vi "Header Names Single.vi"(11 "Dynamic Data":dynamicdata(waveform)) -> (3 "Signals Out":dynamicdata(waveform))   [LabVIEW 2017]
uses:
  <vilib>/express/express shared/transition.llb/Dynamic To Waveform Array.vi
  <vilib>/express/express signal manip/GetorSetDDTAttributes/Set DDT Attributes/SetT0.vi
  <vilib>/express/express shared/transition.llb/Waveform Array To Dynamic.vi
  <vilib>/express/express signal manip/GetorSetDDTAttributes/Set DDT Attributes/Set DDT Properties.xnode
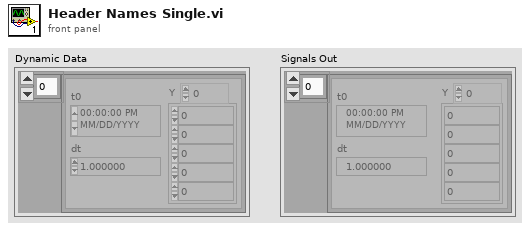
[diagram p1: front panel]
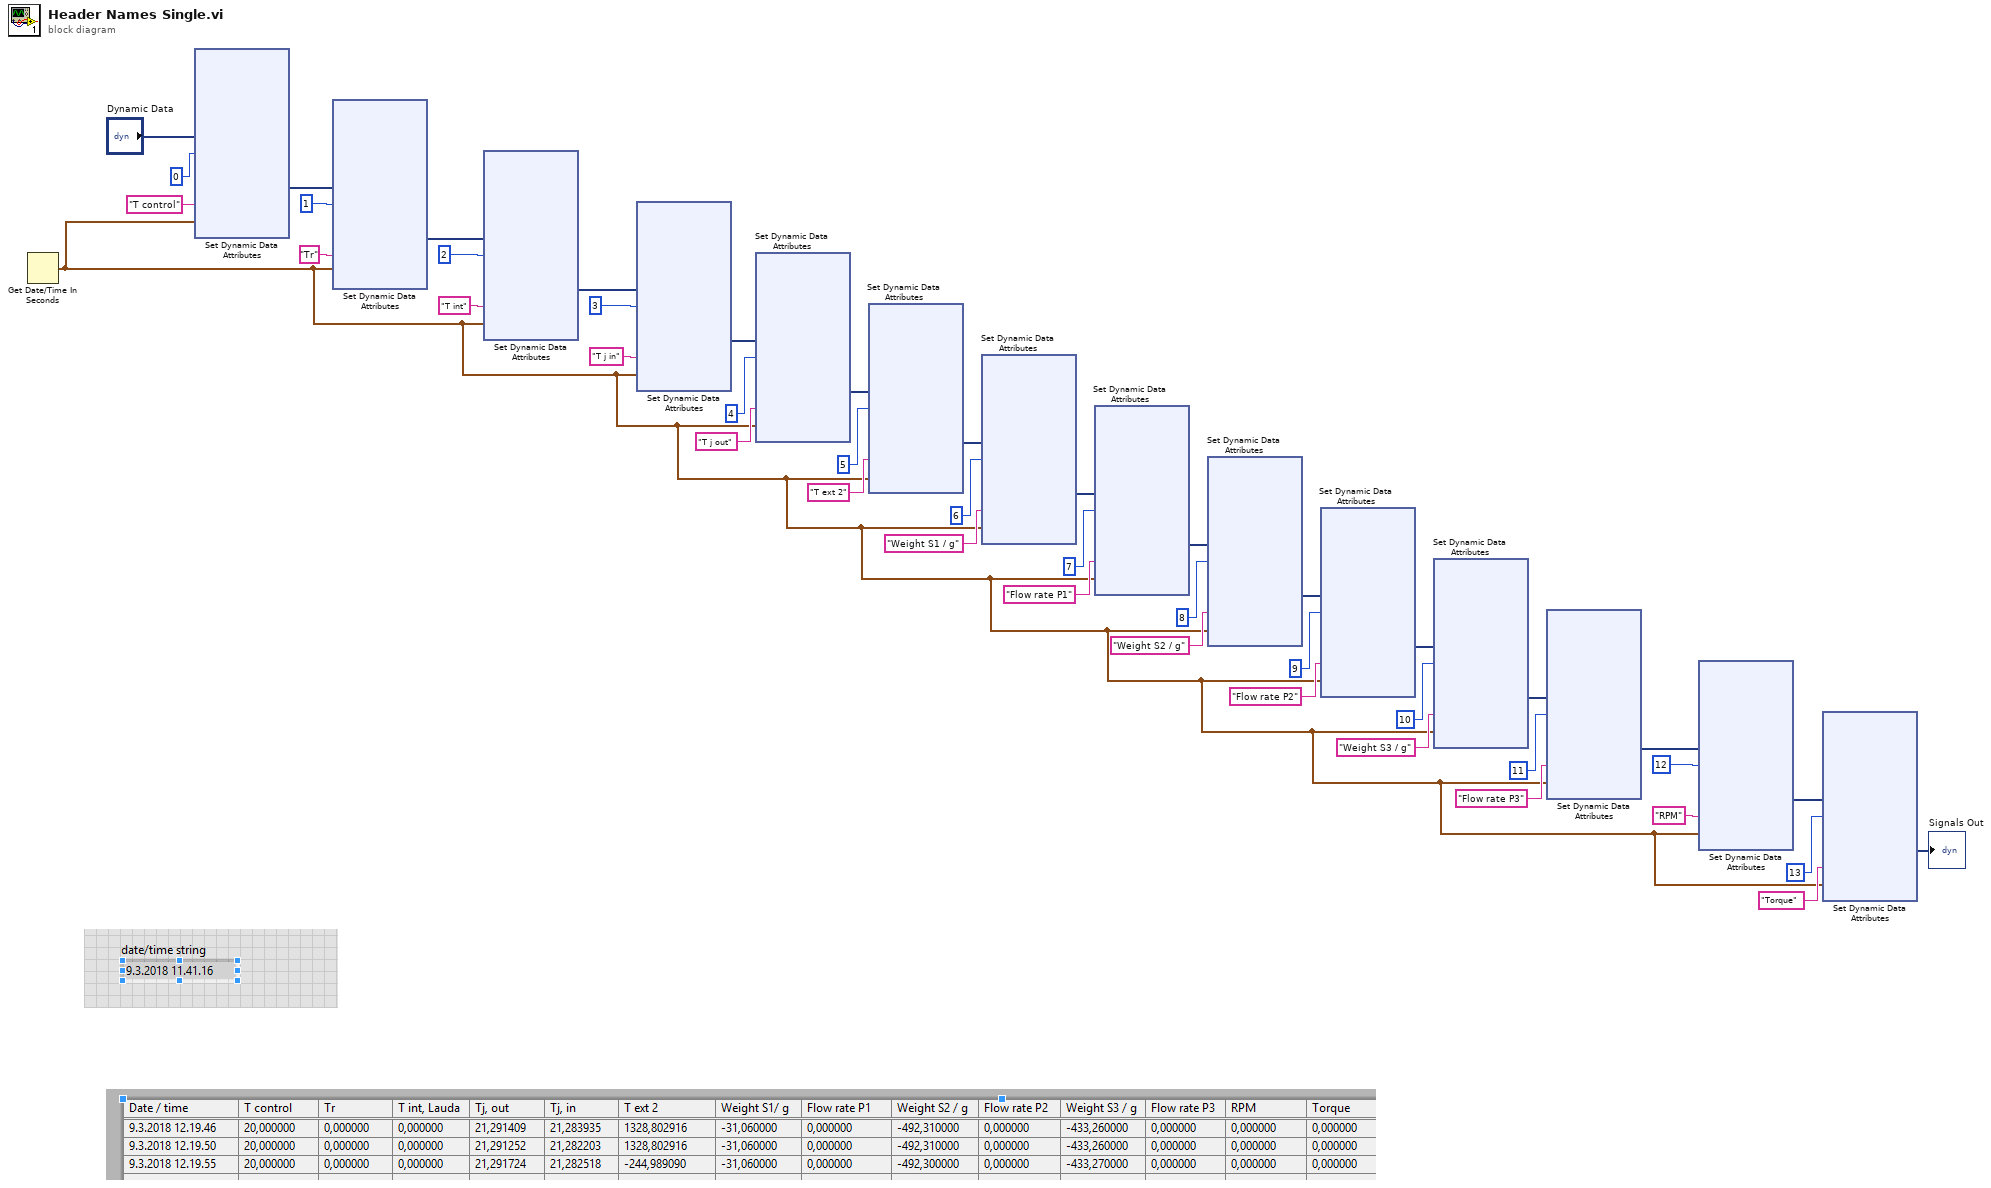
[diagram p0: block diagram]
diagram:
  n1 = Get Date/Time In Seconds() -> (seconds since 1Jan1904=w1:timestamp)
  n2 = xnode "Set Dynamic Data Attributes"("Signals In"="Dynamic Data", "Signal Index"=0, "Signal Name"="T control", "Timestamp"=w1) -> ("Signals Out"=w10:dynamicdata)  [unwired: 1 in, 1 out]
  n3 = xnode "Set Dynamic Data Attributes"("Signals In"=w10, "Signal Index"=1, "Signal Name"="Tr", "Timestamp"=w1) -> ("Signals Out"=w11:dynamicdata)  [unwired: 1 in, 1 out]
  n4 = xnode "Set Dynamic Data Attributes"("Signals In"=w11, "Signal Index"=2, "Signal Name"="T int", "Timestamp"=w1) -> ("Signals Out"=w14:dynamicdata)  [unwired: 1 in, 1 out]
  n5 = xnode "Set Dynamic Data Attributes"("Signals In"=w14, "Signal Index"=3, "Signal Name"="T j in", "Timestamp"=w1) -> ("Signals Out"=w17:dynamicdata)  [unwired: 1 in, 1 out]
  n6 = xnode "Set Dynamic Data Attributes"("Signals In"=w17, "Signal Index"=4, "Signal Name"="T j out", "Timestamp"=w1) -> ("Signals Out"=w20:dynamicdata)  [unwired: 1 in, 1 out]
  n7 = xnode "Set Dynamic Data Attributes"("Signals In"=w20, "Signal Index"=5, "Signal Name"="T ext 2", "Timestamp"=w1) -> ("Signals Out"=w38:dynamicdata)  [unwired: 1 in, 1 out]
  n8 = xnode "Set Dynamic Data Attributes"("Signals In"=w38, "Signal Index"=6, "Signal Name"="Weight S1 / g", "Timestamp"=w1) -> ("Signals Out"=w27:dynamicdata)  [unwired: 1 in, 1 out]
  n9 = xnode "Set Dynamic Data Attributes"("Signals In"=w27, "Signal Index"=7, "Signal Name"="Flow rate P1", "Timestamp"=w1) -> ("Signals Out"=w28:dynamicdata)  [unwired: 1 in, 1 out]
  n10 = xnode "Set Dynamic Data Attributes"("Signals In"=w28, "Signal Index"=8, "Signal Name"="Weight S2 / g", "Timestamp"=w1) -> ("Signals Out"=w31:dynamicdata)  [unwired: 1 in, 1 out]
  n11 = xnode "Set Dynamic Data Attributes"("Signals In"=w31, "Signal Index"=9, "Signal Name"="Flow rate P2", "Timestamp"=w1) -> ("Signals Out"=w34:dynamicdata)  [unwired: 1 in, 1 out]
  n12 = xnode "Set Dynamic Data Attributes"("Signals In"=w34, "Signal Index"=10, "Signal Name"="Weight S3 / g", "Timestamp"=w1) -> ("Signals Out"=w37:dynamicdata)  [unwired: 1 in, 1 out]
  n13 = xnode "Set Dynamic Data Attributes"("Signals In"=w37, "Signal Index"=11, "Signal Name"="Flow rate P3", "Timestamp"=w1) -> ("Signals Out"=w44:dynamicdata)  [unwired: 1 in, 1 out]
  n14 = xnode "Set Dynamic Data Attributes"("Signals In"=w44, "Signal Index"=12, "Signal Name"="RPM", "Timestamp"=w1) -> ("Signals Out"=w43:dynamicdata)  [unwired: 1 in, 1 out]
  n15 = xnode "Set Dynamic Data Attributes"("Signals In"=w43, "Signal Index"=13, "Signal Name"="Torque", "Timestamp"=w1) -> ("Signals Out"=→"Signals Out":dynamicdata)  [unwired: 1 in, 1 out]
